vi "Handle Error.vi"(6 "Current Account":u32, 7 "Command":T1(ring)=enum."Handle", 8 "error in (no error)":errorcluster, 9 "Clear Error?":bool=TRUE, 10 "Classification":T2, 11 "Error Codes":i32[](array[numeric])) -> (0 "error out":errorcluster, 2 "System Error":bool, 3 "Session Error":bool)   [LabVIEW 2012]
doc: "Specifying a non-empty array for Error Codes causes the error to be handled only if it matches on of the error codes. In this mode, warnings are handled the same as errors.\nSpecifying an empty array for Error Code causes the function to handle any error. In this mode, warnings are ignored."
uses:
  TypeDefs/Error Classification.ctl
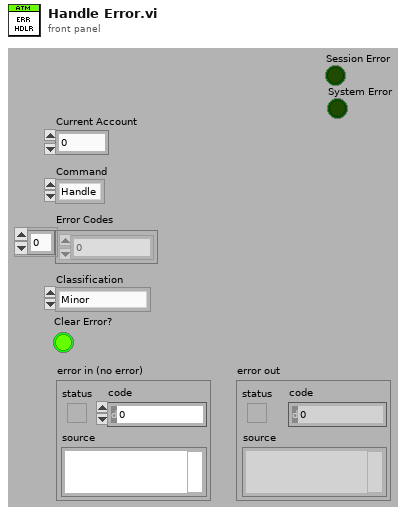
[diagram p1: front panel]
types:
  T1 = enum16{"Init", "Handle", "Check", "Close", "Set Current Account"}
  T2 = typedef "Error Classification.ctl" = enum16{"Minor", "Session", "System"}
  T3 = enum16{"open", "replace", "create", "open or create", "replace or create", "replace or create with confirmation"}
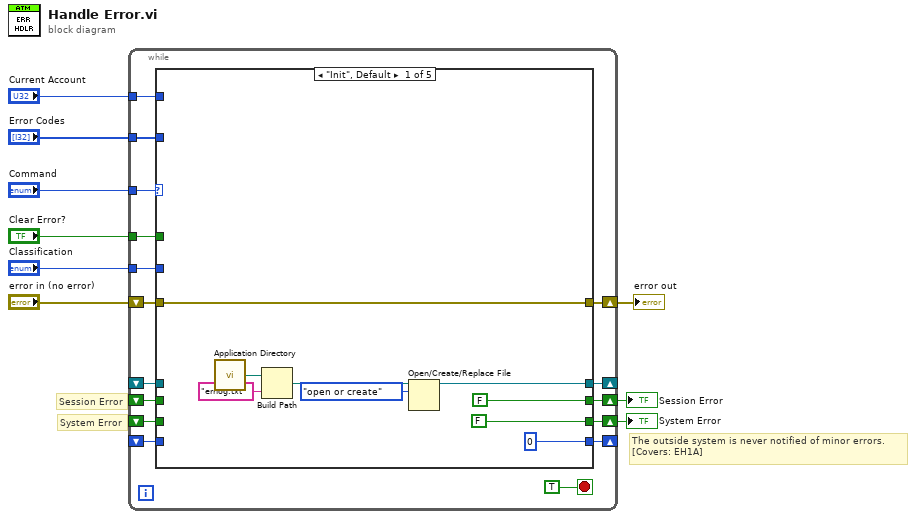
[diagram p0: block diagram]
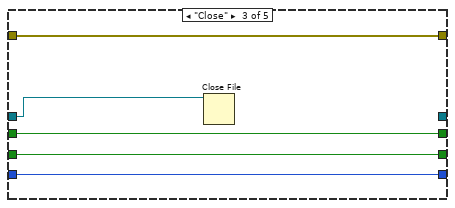
[diagram p3: hidden frame]
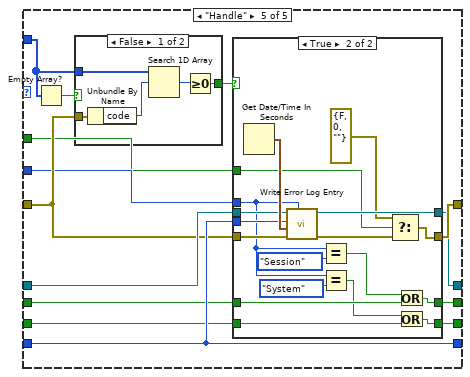
[diagram p5: hidden frame]
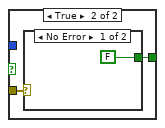
[diagram p7: hidden frame]
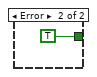
[diagram p8: hidden frame]
diagram:
  # "The outside system is never notified of minor errors.\n[Covers: EH1A]"
  # "System Error"
  # "Session Error"
  n1 = while {
    tunnel: "Command" -> [w24]
    shift-right: [w23] -> w3
    shift-left: _ -> [w22]
    shift-right: [w21] -> w2
    shift-left: _ -> [w20]
    shift-right: [w17] -> w6
    shift-left: "error in (no error)" -> [w19]
    tunnel: "Error Codes" -> [w18]
    shift-right: [w16] -> _
    shift-left: _ -> [w15]
    shift-right: [w14] -> _
    shift-left: _ -> [w13]
    tunnel: "Classification" -> [w12]
    tunnel: "Clear Error?" -> [w11]
    tunnel: "Current Account" -> [w10]
    stop <- TRUE stop-if-true
    n2 = case shown="\"Init\", Default" w24 {
      tunnel: [FALSE ("Session Error") w39 w44 w49 w50] -> w23
      tunnel: w22 -> [_ w39 w44 w49 w53]
      tunnel: [FALSE ("System Error") w38 w43 w48 w51] -> w21
      tunnel: w20 -> [_ w38 w43 w48 w52]
      tunnel: w19 -> [w32 w37 w42 w47 w58]
      tunnel: w18 -> [_ _ _ _ w62]
      tunnel: [w32 w37 w42 w47 w57] -> w17
      tunnel: [u32 0 w36 w41 w45 w59] -> w16
      tunnel: w15 -> [_ w36 w41 _ w59]
      tunnel: [w30 w35 _ w46 w54] -> w14
      tunnel: w13 -> [_ w35 w40 w46 w60]
      tunnel: w12 -> [_ _ _ _ w56]
      tunnel: w11 -> [_ _ _ _ w55]
      tunnel: w10 -> [_ _ _ w45 _]
      frame "Init", Default {
        n3 = call <vilib>:"Application Directory.vi"() -> ("Application Directory"=w29:path)
        n4 = Build Path(base path=w29, name or relative path="errlog.txt") -> (appended path=w28:path)
        n5 = Open/Create/Replace File(file path (use dialog)=w28, operation (0:open)=T3."open or create") -> (refnum out=w30:refnum<file>)  [unwired: 4 in, 2 out]
      }
      frame "Check" {
      }
      frame "Close" {
        n6 = Close File(refnum=w40) -> ()  [unwired: 1 in, 2 out]
      }
      frame "Set Current Account" {
      }
      frame "Handle" {
        n7 = Empty Array?(array=w62) -> (empty?=w63:bool)
        n8 = case shown="False" w63 {
          tunnel: w58 -> [w90 w92]
          tunnel: w62 -> [w89 _]
          tunnel: [w86 w91] -> w61
          frame False {
            n9 = Unbundle By Name(w90) -> ("code"=w88:i32)
            n10 = Search 1D Array(1D array=w89, element=w88) -> (index of element=w87:i32)  [unwired: 1 in]
            n11 = Greater Or Equal To 0?(x=w87) -> (x >= 0?=w86:bool)
          }
          frame True {
            n12 = case shown="No Error" w92 {
              tunnel: [FALSE TRUE] -> w91
              frame No Error {
              }
              frame Error {
              }
            }
          }
        }
        n13 = case shown="True" w61 {
          tunnel: w60 -> [w64 w84]
          tunnel: w59 -> [_ w83]
          tunnel: w58 -> [w67 w82]
          tunnel: [w67 w70] -> w57
          tunnel: w56 -> [_ w73]
          tunnel: w55 -> [_ w69]
          tunnel: [w64 w81] -> w54
          tunnel: w53 -> [w66 w78]
          tunnel: w52 -> [w65 w80]
          tunnel: [w65 w79] -> w51
          tunnel: [w66 w77] -> w50
          frame False {
          }
          frame True {
            n14 = Get Date/Time In Seconds() -> (seconds since 1Jan1904=w85:timestamp)
            n15 = call "Write Error Log Entry.vi"("Classification"=w73, "error in (no error)"=w82, "current time"=w85, "Account #"=w83, "Log Ref In"=w84) -> ("error out"=w71:errorcluster, "Log Ref Out"=w81:refnum<file>)  [unwired: 5 in]
            n16 = Equal?(x=w73, y=Error_Classification."Session") -> (x = y?=w74:bool)
            n17 = Equal?(x=w73, y=Error_Classification."System") -> (x = y?=w72:bool)
            n18 = Select(t=errorcluster {"status"=FALSE, "code"=0, "source"=""}, s=w69, f=w71) -> (s? t:f=w70:errorcluster)
            n19 = Or(x=w74, y=w78) -> (x .or. y?=w77:bool)
            n20 = Or(x=w72, y=w80) -> (x .or. y?=w79:bool)
          }
        }
      }
    }
  }
  "error out" <- w6
  "Session Error" <- w3
  "System Error" <- w2
